vi "Setup UI.vi"(8 "error in (no error)":errorcluster, 10 "Set UI to input? (F)":bool, 11 "LCD Reader in":refnum<class "LCD Reader.lvclass">) -> (0 "error out":errorcluster, 3 "LCD Reader out":refnum<class "LCD Reader.lvclass">)   [LabVIEW 2009, in "LCD Reader.lvclass"]
doc: "Setup UI constructs an object -- populates its member data -- from a front panel the user can see. The VI should be as simple as possible so that a UI loop can poll it continuously for updates. \n\nThe VI is designed to be used as a subPanel within another VI. Wire true to \"Set UI to input\" only on the first call, just after inserting this VI into a subPanel, to populate its controls with the class's current values.\n\nSetup UI is distinct from the class constructor. Class constructors are not polymorphic, yet configure dialogs need to configure objects without knowing their type -- and polymorphism is the necessary solution. Thus, Setup UI is a polymorphic class constructor. This continously polled \"Setup UI\" concept is a kludge: a better idea would be an XControl, but those require a steeper learning curve."
uses:
  LCD Reader.lvclass
  LCD Reader.lvclass/LCD Reader.ctl
  Reader/Reader.lvclass
panel:
  in  "?":bool
  in  "LCD 1/4 Wave Retardance":dbl[unit]
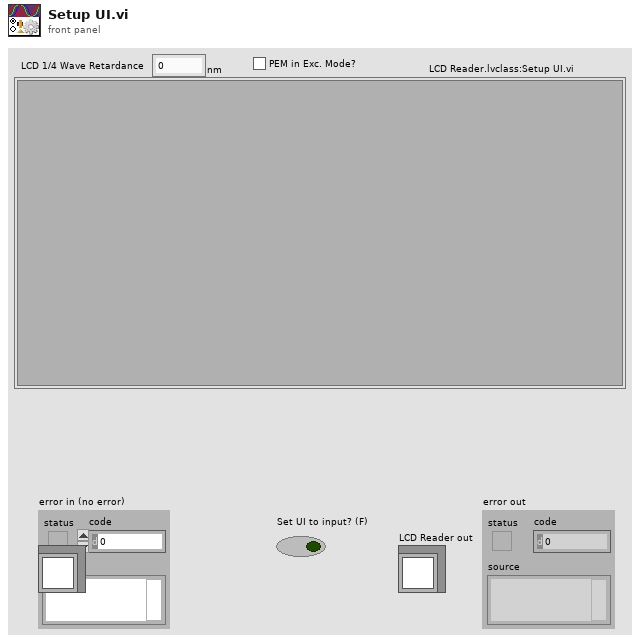
[diagram p1: front panel]
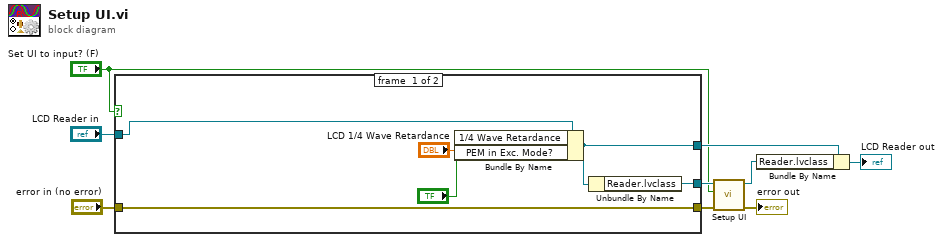
[diagram p0: block diagram]
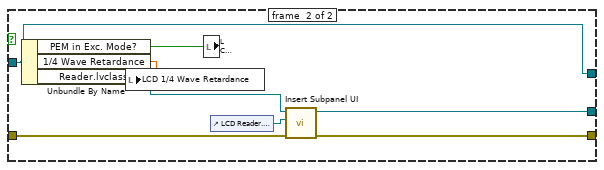
[diagram p2: hidden frame]
diagram:
  n1 = case shown="False" "Set UI to input? (F)" {
    tunnel: "error in (no error)" -> [w15 w23]
    tunnel: [w15 w22] -> w3
    tunnel: "LCD Reader in" -> [w14 w16]
    tunnel: [w11 w16] -> w7
    tunnel: [w10 w17] -> w4
    frame #0 {
      n2 = Bundle By Name(cluster=w14, "1/4 Wave Retardance"="LCD 1/4 Wave Retardance", "PEM in Exc. Mode?"="?") -> (w11:refnum<class "LCD Reader.lvclass">)
      n3 = Unbundle By Name(w11) -> ("Reader.lvclass"=w10:refnum<class "Reader.lvclass">)
    }
    frame #1 {
      n4 = Unbundle By Name(w16) -> ("PEM in Exc. Mode?"=w21:bool, "1/4 Wave Retardance"=w20:dbl[unit], "Reader.lvclass"=w19:refnum<class "Reader.lvclass">)
      n5 = local write "LCD 1/4 Wave Retardance"(w20) -> ()
      n6 = local write item#6(w21) -> ()
      n7 = control-ref of="LCD Reader.lvclass:Setup UI.vi"() -> (w18:refnum<vi>)
      n8 = call "Insert Subpanel UI.vi"("error in (no error)"=w23, "Subpanel in"=w18, "LabVIEW Object"=w19) -> ("error out"=w22:errorcluster, "LabVIEW Object out"=w17:refnum<class "Reader.lvclass">)  [unwired: 7 out]
    }
  }
  n9 = call-dynamic "Setup UI.vi"("error in (no error)"=w3, "Set UI to input? (F)"="Set UI to input? (F)", "Reader in"=w4) -> ("error out"=→"error out":errorcluster, "Reader out"=w5:refnum<class "Reader.lvclass">)  [unwired: 7 out]
  n10 = Bundle By Name(cluster=w7, "Reader.lvclass"=w5) -> (→"LCD Reader out":refnum<class "LCD Reader.lvclass">)
